vi "Mean.vi"(1 "Array":dbl[](array[numeric])) -> (0 "Mean":dbl)   [LabVIEW 2020, in "Endigit.lvlib"]
doc: "Performs a mean calculation much more efficiently than the LabVIEW primitive. Returns 0 if the array is empty.\n\nAuthored by Robert C. Mortensen\nrobert@endigit.com\n\nCopyright (c) 2015, Endigit, Inc."
uses:
  Endigit.lvlib
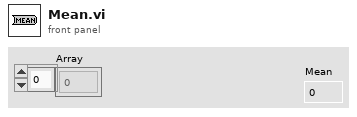
[diagram p1: front panel]
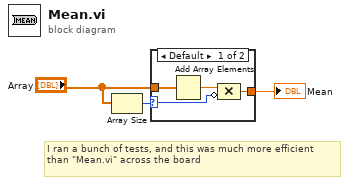
[diagram p0: block diagram]
diagram:
  # "I ran a bunch of tests, and this was much more efficient than \"Mean.vi\" across the board"
  n1 = Array Size(array="Array") -> (size(s)=w3:i32)
  n2 = case shown="Default" w3 {
    selector: w3 -> [w6 _]
    tunnel: "Array" -> [w7 _]
    tunnel: [w5 _] -> w1
    frame Default {
      n3 = Add Array Elements(numeric array=w7) -> (sum=w4:dbl)
      n4 = Compound Arithmetic op=MULTIPLY(w4, invert w6) -> (w5:dbl)
    }
    frame 0 {
    }
  }
  "Mean" <- w1
